vi "acknowledgeIRQ.vi"(8 "error in (no error)":errorcluster, 10 "IRQs":i32[](array[numeric]), 11 "ModbusIRQ in":refnum<class "ModbusIRQ.lvclass">) -> (0 "error out":errorcluster, 3 "ModbusIRQ out":refnum<class "ModbusIRQ.lvclass">)   [LabVIEW 2016, in "ModbusIRQ.lvclass"]
uses:
  ModbusIRQ.lvclass
  ModbusIRQ.lvclass/ModbusIRQ.ctl
  FPGA/FPGA.lvclass
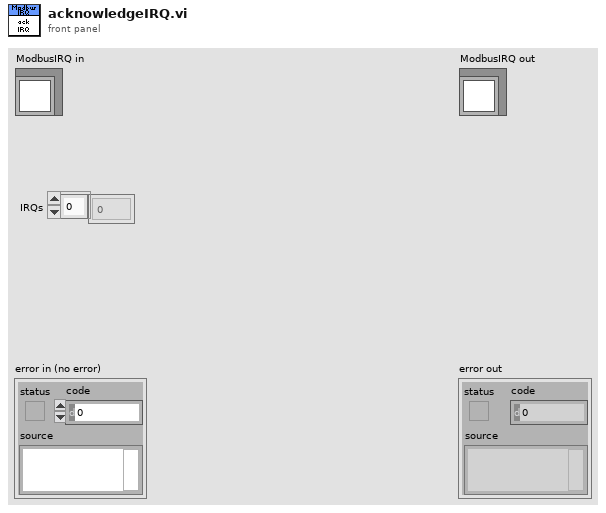
[diagram p1: front panel]
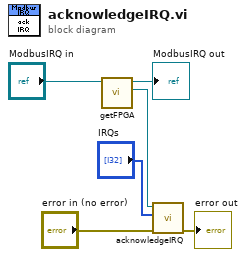
[diagram p0: block diagram]
diagram:
  n1 = call "getFPGA.vi"("ModbusIRQ in"="ModbusIRQ in") -> ("FPGA"=w5:refnum<class "FPGA.lvclass">, "ModbusIRQ out"=→"ModbusIRQ out":refnum<class "ModbusIRQ.lvclass">)  [unwired: 9 in]
  n2 = call "acknowledgeIRQ.vi"("error in (no error)"="error in (no error)", "IRQs"="IRQs", "FPGA in"=w5) -> ("error out"=→"error out":errorcluster)  [unwired: 7 in, 1 out]
